vi "Spectrum Unit Conversion.vi"(4 "window constants":cluster{"eq noise BW":dbl, "coherent gain":dbl}={"eq noise BW"=1.0, "coherent gain"=1.0} {"coherent gain" format="%0.2f"; "eq noise BW" format="%0.2f"}, 6 "df":dbl=1.0 format="%0.2f", 7 "signal unit (V)":string="V", 8 "display unit":T2(ring), 9 "log/linear":enum16{"Linear", "dB", "dBm"}(ring)=enum."dB", 10 "spectrum type":T1(ring), 11 "Spectrum in":dbl[](array[numeric])) -> (0 "spectrum unit":string="dBVrms", 3 "Spectrum out":dbl[](array[numeric]))   [LabVIEW 2017, in "NI_AALPro.lvlib"]
doc: "Converts either the power, amplitude, or gain (amplitude ratio) spectrum to alternate formats including Log (decibel and dbm) and spectral density."
uses:
  NI_AALPro.lvlib
panel:
  # "Spectrum Unit Conversion"
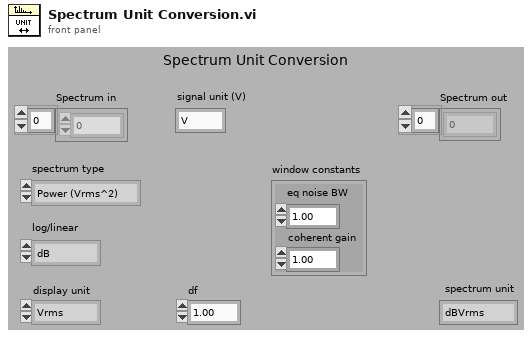
[diagram p1: front panel]
types:
  T1 = enum16{"Power (Vrms^2)", "Amplitude (Vrms)", "Gain (amplitude ratio)"}
  T2 = enum32{"Vrms", "Vpk", "Vrms^2", "Vpk^2", "Vrms/rtHz", "Vpk/rtHz", "Vrms^2/Hz", "Vpk^2/Hz"}
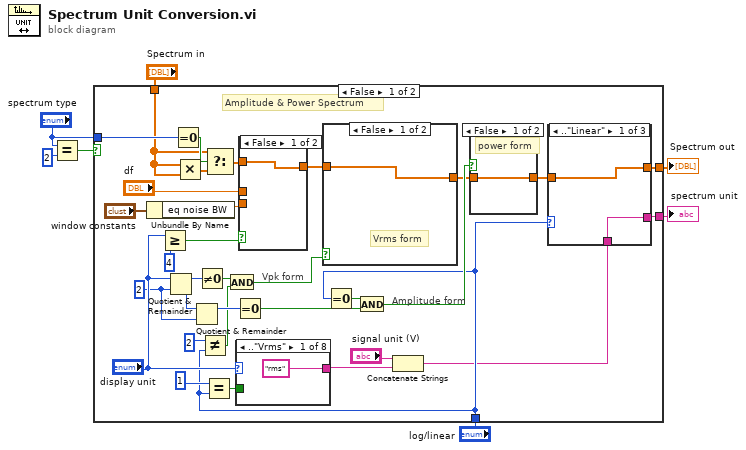
[diagram p0: block diagram]
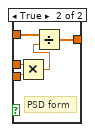
[diagram p2: hidden frame]
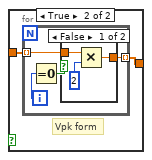
[diagram p3: hidden frame]
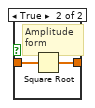
[diagram p5: hidden frame]
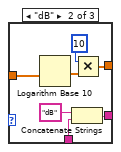
[diagram p6: hidden frame]
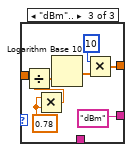
[diagram p7: hidden frame]
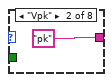
[diagram p8: hidden frame]
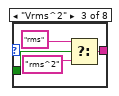
[diagram p9: hidden frame]
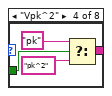
[diagram p10: hidden frame]
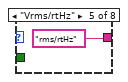
[diagram p11: hidden frame]
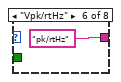
[diagram p12: hidden frame]
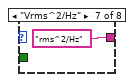
[diagram p13: hidden frame]
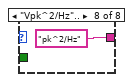
[diagram p14: hidden frame]
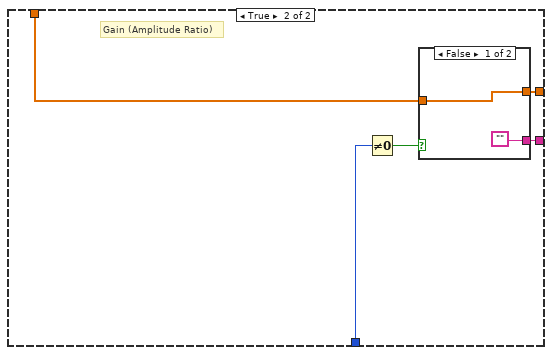
[diagram p15: hidden frame]
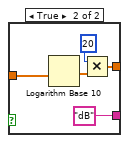
[diagram p16: hidden frame]
diagram:
  n1 = Equal?(x="spectrum type", y=2) -> (x = y?=w6:bool)
  n2 = case shown="False" w6 {
    tunnel: [w24 w96] -> w7
    tunnel: [w23 w95] -> w1
    tunnel: "spectrum type" -> [w21 _]
    tunnel: "Spectrum in" -> [w20 w94]
    tunnel: "log/linear" -> [w15 w92]
    frame False {
      w34 = 2
      # "Amplitude & Power Spectrum"
      # "Vpk form"
      # "Amplitude form"
      n3 = Unbundle By Name("window constants") -> ("eq noise BW"=w30:dbl)
      n4 = Greater Or Equal?(x="display unit", y=4) -> (x >= y?=w28:bool)
      n5 = Quotient & Remainder(x="display unit", y=w34) -> (x-y*floor(x/y)=w31:u32, floor(x/y)=w33:u32)
      n6 = Equal To 0?(x=w21) -> (x = 0?=w25:bool)
      n7 = Multiply(x=w20, y=w20) -> (x*y=w26:dbl[])
      n8 = Quotient & Remainder(x=w33, y=w34) -> (x-y*floor(x/y)=w35:u32)  [unwired: 1 out]
      n9 = Not Equal To 0?(x=w31) -> (x != 0?=w13:bool)
      n10 = Not Equal?(x=2, y=w15) -> (x != y?=w14:bool)
      n11 = Equal?(x=1, y=w15) -> (x = y?=w18:bool)
      n12 = Select(t=w20, s=w25, f=w26) -> (s? t:f=w29:dbl[])
      n13 = And(x=w13, y=w14) -> (x .and. y?=w12:bool)
      n14 = Equal To 0?(x=w35) -> (x = 0?=w17:bool)
      n15 = case shown="..\"Vrms\"" "display unit" {
        tunnel: ["rms" "pk" w83 w87 "rms/rtHz" "pk/rtHz" "rms^2/Hz" "pk^2/Hz"] -> w10
        tunnel: w18 -> [_ _ w82 w86 _ _ _ _]
        frame .."Vrms" {
        }
        frame "Vpk" {
        }
        frame "Vrms^2" {
          n16 = Select(t="rms", s=w82, f="rms^2") -> (s? t:f=w83:string)
        }
        frame "Vpk^2" {
          n17 = Select(t="pk", s=w86, f="pk^2") -> (s? t:f=w87:string)
        }
        frame "Vrms/rtHz" {
        }
        frame "Vpk/rtHz" {
        }
        frame "Vrms^2/Hz" {
        }
        frame "Vpk^2/Hz".. {
        }
      }
      n18 = case shown="False" w28 {
        tunnel: [w41 w45] -> w32
        tunnel: w30 -> [_ w44]
        tunnel: w29 -> [w41 w46]
        tunnel: "df" -> [_ w43]
        frame False {
        }
        frame True {
          # "PSD form"
          n19 = Multiply(x=w43, y=w44) -> (x*y=w42:dbl)
          n20 = Divide(x=w46, y=w42) -> (x/y=w45:dbl[])
        }
      }
      n21 = case shown="False" w12 {
        tunnel: [w47 w48] -> w36
        tunnel: w32 -> [w47 w49]
        frame False {
          # "Vrms form"
        }
        frame True {
          # "Vpk form"
          n22 = for {
            tunnel: [w50] -> w48 mode=indexing
            tunnel: w49 -> [w51] mode=indexing
            i -> [w53]
            n23 = Equal To 0?(x=w53) -> (x = 0?=w52:bool)
            n24 = case shown="False" w52 {
              tunnel: [w54 w57] -> w50
              tunnel: w51 -> [w56 w57]
              frame False {
                n25 = Multiply(x=w56, y=2) -> (x*y=w54:dbl)
              }
              frame True {
              }
            }
          }
        }
      }
      n26 = Equal To 0?(x=w15) -> (x = 0?=w40:bool)
      n27 = And(x=w40, y=w17) -> (x .and. y?=w39:bool)
      n28 = Concatenate Strings("signal unit (V)", w10) -> (w9:string)
      n29 = case shown="False" w39 {
        tunnel: [w58 w59] -> w37
        tunnel: w36 -> [w58 w60]
        frame False {
          # "power form"
        }
        frame True {
          # "Amplitude \nform"
          n30 = Square Root(x=w60) -> (sqrt(x)=w59:dbl[])
        }
      }
      n31 = case shown="..\"Linear\"" w15 {
        tunnel: w37 -> [w61 w69 w73]
        tunnel: w9 -> [w62 w65 _]
        tunnel: [w62 w64 "dBm"] -> w23
        tunnel: [w61 w63 w75] -> w24
        frame .."Linear" {
        }
        frame "dB" {
          n32 = Logarithm Base 10(1:w69) -> (0:w68:dbl[])
          n33 = Concatenate Strings("dB", w65) -> (w64:string)
          n34 = Multiply(x=10, y=w68) -> (x*y=w63:dbl[])
        }
        frame "dBm".. {
          w71 = 0.78
          n35 = Multiply(x=w71, y=w71) -> (x*y=w70:dbl)
          n36 = Divide(x=w73, y=w70) -> (x/y=w74:dbl[])
          n37 = Logarithm Base 10(1:w74) -> (0:w77:dbl[])
          n38 = Multiply(x=10, y=w77) -> (x*y=w75:dbl[])
        }
      }
    }
    frame True {
      # "Gain (Amplitude Ratio)"
      n39 = Not Equal To 0?(x=w92) -> (x != 0?=w93:bool)
      n40 = case shown="False" w93 {
        tunnel: [w98 w99] -> w96
        tunnel: w94 -> [w98 w103]
        tunnel: ["" "dB"] -> w95
        frame False {
        }
        frame True {
          n41 = Logarithm Base 10(1:w103) -> (0:w102:dbl[])
          n42 = Multiply(x=20, y=w102) -> (x*y=w99:dbl[])
        }
      }
    }
  }
  "spectrum unit" <- w1
  "Spectrum out" <- w7
